vi "Program.vi"() -> ()   [LabVIEW 2014]
panel:
  in  "stop":bool
  out "error out":errorcluster
  in  "error in (no error)":errorcluster
  in  "设置":bool
  out "转速方向":bool
  out "转矩方向":bool
  in  "停机":bool
  out "欠压":bool
  out "过压":bool
  out "过流":bool
  out "过速":bool
  out "模块过温":bool
  out "电机过温":bool
  out "开关错误":bool
  out "模块故障":bool
  out "String":string
  in  "参数3":dbl
  in  "参数2":dbl
  in  "参数1":dbl
  in  "指令名":dbl
  in  "发送":bool
  in  "录波?L":bool caption="录波"
  out "波形文件大小L":string
  out "已录波L":string
  out "录波开始时间L":string
  in  "模式选择L":u16(ring) items=["示波模式", "录波模式", "XY图模式"]
  out "XY Graph L":cluster{"Y":dbl[], "Y":dbl[]}[](graph)
  in  "Choose 2":u16(ring) items=["Estlalpha", "AlphaErr", "speed", "iq", "id"]
  in  "Choose 1":u16(ring) items=["Estlalpha", "AlphaErr", "speed", "iq", "id"]
  in  "时频域转换 2":bool
  out "Graph 2":dbl[](graph)
  in  "时频域转换 1":bool
  out "Graph 1":dbl[](graph)
  in  "录波?R":bool caption="录波"
  out "波形文件大小R":string
  out "已录波R":string
  out "录波开始时间R":string
  in  "模式选择R":u16(ring) items=["示波模式", "录波模式", "XY图模式"]
  out "XY Graph R":cluster{"Y":dbl[], "Y":dbl[]}[](graph)
  in  "Choose 4":u16(ring) items=["Estlalpha", "AlphaErr", "speed", "iq", "id"]
  in  "Choose 3":u16(ring) items=["Estlalpha", "AlphaErr", "speed", "iq", "id"]
  in  "时频域转换 4":bool
  out "Graph 4":dbl[](graph)
  in  "时频域转换 3":bool
  out "Graph 3":dbl[](graph)
  # "电机工作状态"
  # "电机故障状态"
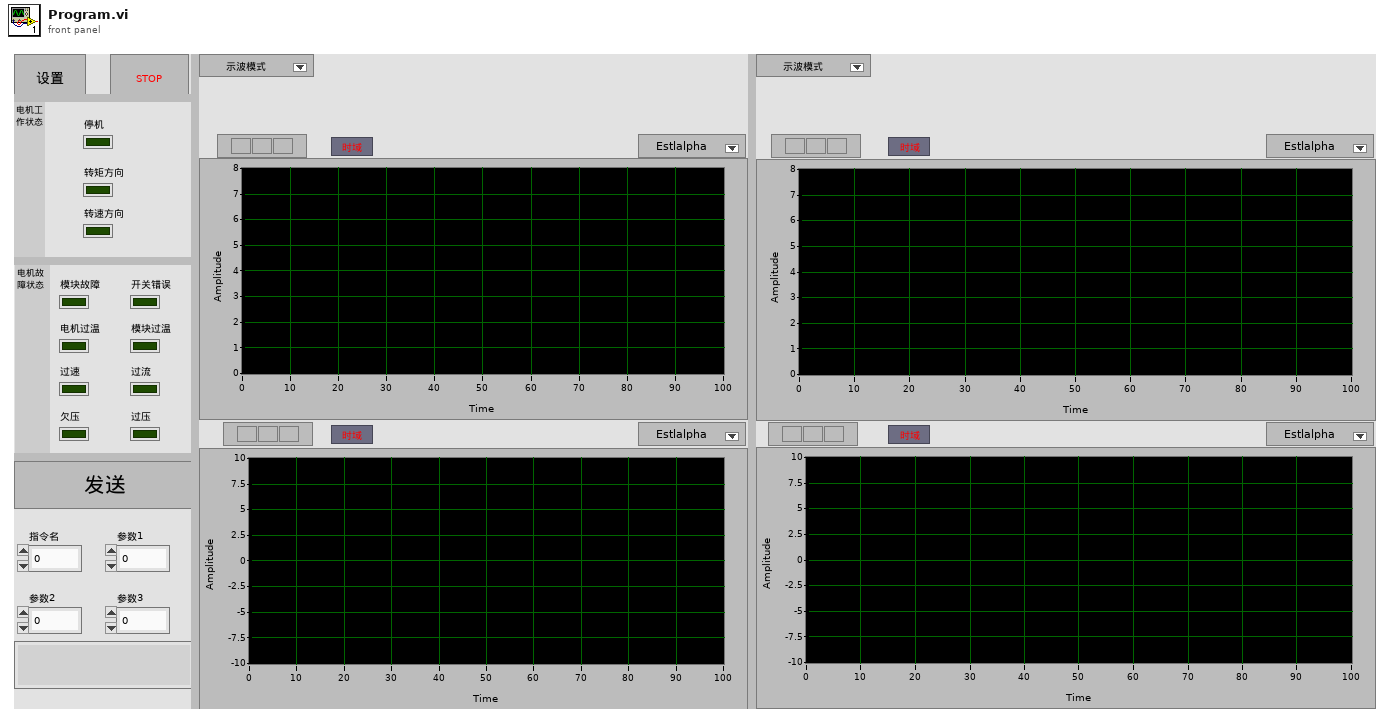
[diagram p1: front panel]
types:
  T1 = cluster{"ID":u32, "TimeStamp":u32, "TimeFlag":u8, "SendType":u8, "RemoteFlag":u8, "ExternFlag":u8, "DataLen":u8, "Data 0":u8, "Data 1":u8, "Data 2":u8, "Data 3":u8, "Data 4":u8, "Data 5":u8, "Data 6":u8, "Data 7":u8, "Reserved 0":u8, "Reserved 1":u8, "Reserved 2":u8}
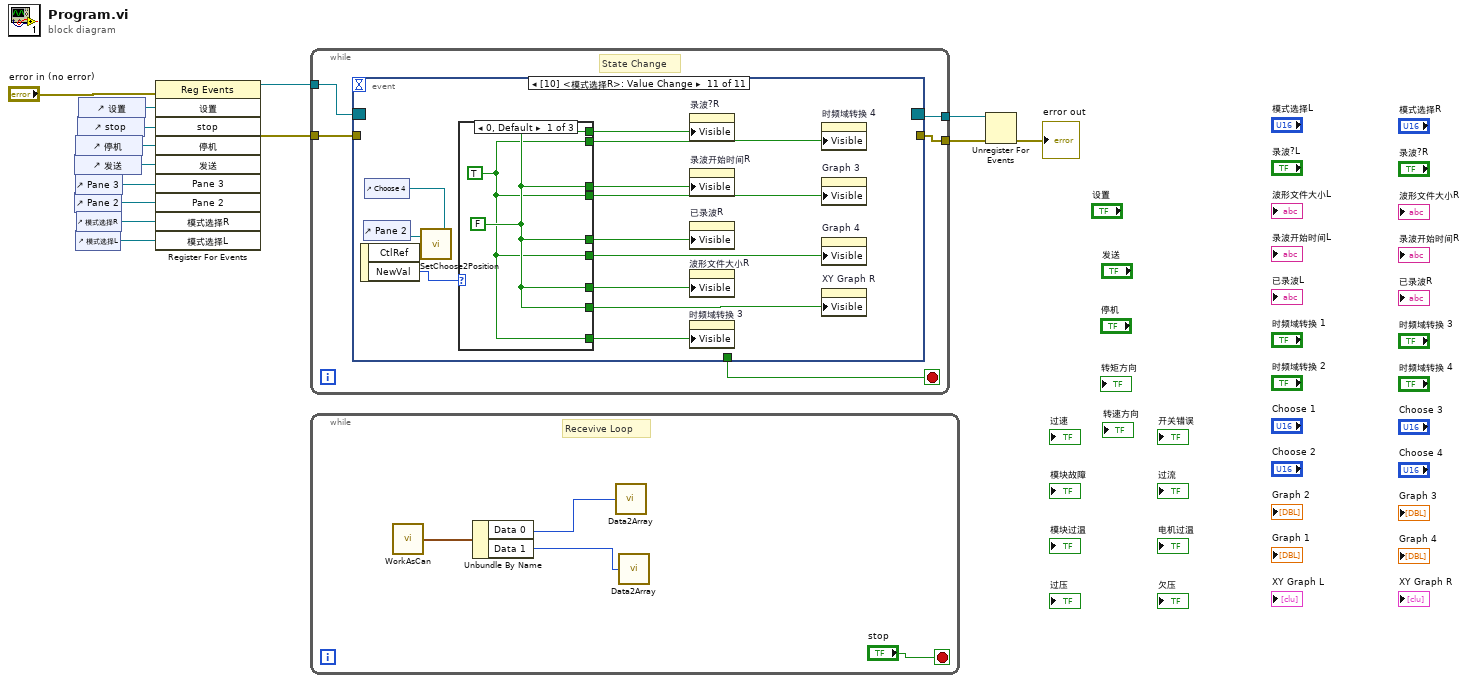
[diagram p0: block diagram]
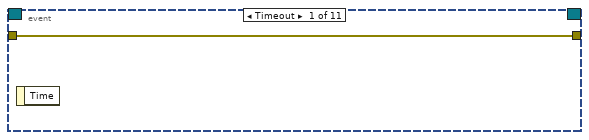
[diagram p2: hidden frame]
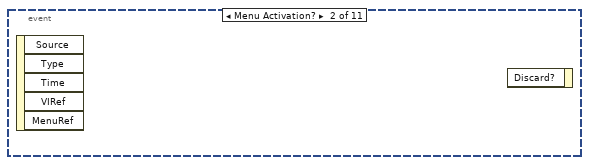
[diagram p3: hidden frame]
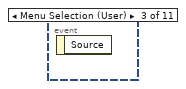
[diagram p4: hidden frame]
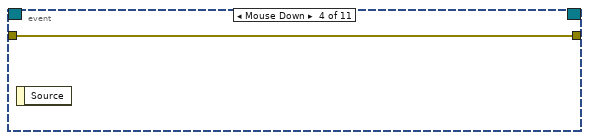
[diagram p5: hidden frame]
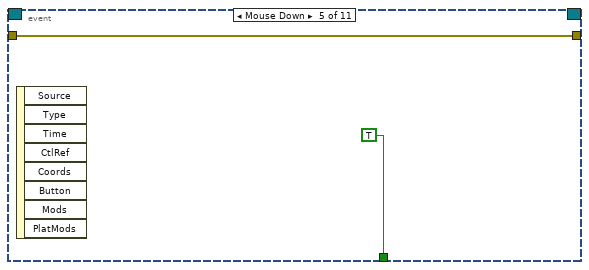
[diagram p6: hidden frame]
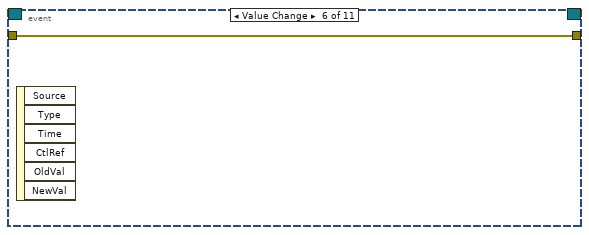
[diagram p7: hidden frame]
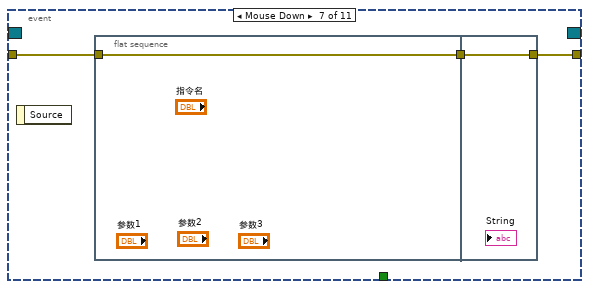
[diagram p8: hidden frame]
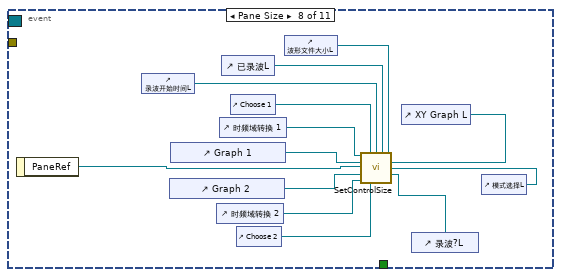
[diagram p9: hidden frame]
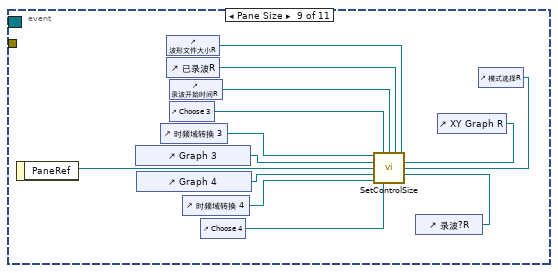
[diagram p10: hidden frame]
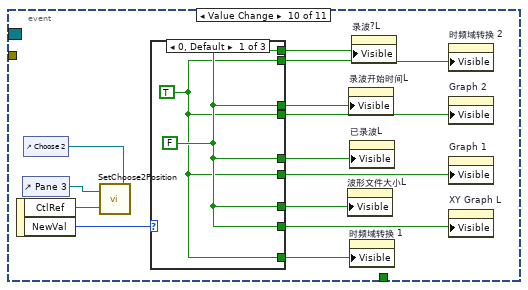
[diagram p11: hidden frame]
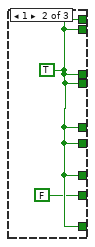
[diagram p12: hidden frame]
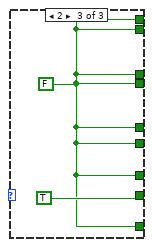
[diagram p13: hidden frame]
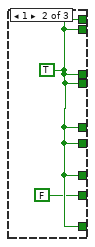
[diagram p14: hidden frame]
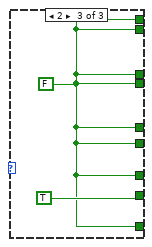
[diagram p15: hidden frame]
diagram:
  n1 = control-ref of="发送"() -> (w10:refnum<vi>)
  n2 = control-ref of="Pane 2"() -> (w3:refnum<vi>)
  n3 = control-ref of="停机"() -> (w11:refnum<vi>)
  n4 = control-ref of="Pane 3"() -> (w4:refnum<vi>)
  n5 = control-ref of="模式选择L"() -> (w1:refnum<vi>)
  n6 = control-ref of="模式选择R"() -> (w2:refnum<vi>)
  n7 = control-ref of="stop"() -> (w5:refnum<vi>)
  n8 = control-ref of="设置"() -> (w14:refnum<vi>)
  n9 = register-events(error in="error in (no error)", w14, w5, w11, w10, w4, w3, w2, w1) -> (reference out=w13:refnum<event-registration>, error out=w8:errorcluster)  [unwired: 1 in]
  n10 = while {
    tunnel: w13 -> [w19]
    tunnel: [w18] -> w12
    tunnel: w8 -> [w16]
    tunnel: [w15] -> w7
    stop <- w17 stop-if-true
    # "State Change"
    n11 = event shown="[10] <模式选择R>: Value Change" {
      selector: w19 -> [_ _ _ _ _ _ _ _ _ _ _]
      dyn-events: [_ _ _ _ _ _ _ _ _ _ _] -> w18
      timeout: _ -> [_ _ _ _ _ _ _ _ _ _ _]
      tunnel: [_ _ _ _ TRUE _ _ _ _ _ _] -> w17
      tunnel: w16 -> [w20 _ _ w21 w22 w24 w27 _ _ _ _]
      tunnel: [w20 _ _ w21 w22 w24 w25 _ _ _ _] -> w15
      event Timeout {
        n12 = event-data() -> ()  [unwired: 1 in, 1 out]
      }
      event Menu Activation? {
        n13 = event-data() -> ()  [unwired: 1 in, 5 out]
        n14 = event-data() -> ()  [unwired: 2 in, 1 out]
      }
      event Menu Selection (User) {
        n15 = event-data() -> ()  [unwired: 1 in, 1 out]
      }
      event Mouse Down {
        n16 = event-data() -> ()  [unwired: 1 in, 1 out]
      }
      event Mouse Down {
        n17 = event-data() -> ()  [unwired: 1 in, 8 out]
      }
      event Value Change {
        n18 = event-data() -> ()  [unwired: 1 in, 6 out]
      }
      event Mouse Down {
        n19 = event-data() -> ()  [unwired: 1 in, 1 out]
        n20 = flat-sequence {
          tunnel: w27 -> [w28]
          tunnel: [w28] -> w26
          tunnel: w26 -> [w29]
          tunnel: [w29] -> w25
          frame #0 {
          }
          frame #1 {
          }
        }
      }
      event Pane Size {
        n21 = event-data() -> ("PaneRef"=w31:refnum<vi>)  [unwired: 1 in]
        n22 = control-ref of="录波开始时间L"() -> (w36:refnum<vi>)
        n23 = control-ref of="Graph 2"() -> (w41:refnum<vi>)
        n24 = control-ref of="Graph 1"() -> (w42:refnum<vi>)
        n25 = control-ref of="时频域转换 2"() -> (w40:refnum<vi>)
        n26 = control-ref of="时频域转换 1"() -> (w39:refnum<vi>)
        n27 = control-ref of="已录波L"() -> (w35:refnum<vi>)
        n28 = control-ref of="Choose 1"() -> (w37:refnum<vi>)
        n29 = control-ref of="Choose 2"() -> (w38:refnum<vi>)
        n30 = control-ref of="波形文件大小L"() -> (w34:refnum<vi>)
        n31 = control-ref of="XY Graph L"() -> (w32:refnum<vi>)
        n32 = control-ref of="录波?L"() -> (w33:refnum<vi>)
        n33 = control-ref of="模式选择L"() -> (w30:refnum<vi>)
        n34 = call "SetControlSize.vi"("时频域1"=w39, "Choose1"=w37, "录波开始时间"=w36, "已录波"=w35, "录波文件大小"=w34, "Graph1"=w42, "XYGraph"=w32, "Pane Refnum"=w31, "Mode"=w30, "Graph2"=w41, "录波？"=w33, "时频域2"=w40, "Choose2"=w38) -> ()  [unwired: 3 in]
      }
      event Pane Size {
        n35 = event-data() -> ("PaneRef"=w55:refnum<vi>)  [unwired: 1 in]
        n36 = control-ref of="Graph 3"() -> (w54:refnum<vi>)
        n37 = control-ref of="Graph 4"() -> (w53:refnum<vi>)
        n38 = control-ref of="时频域转换 3"() -> (w51:refnum<vi>)
        n39 = control-ref of="波形文件大小R"() -> (w46:refnum<vi>)
        n40 = control-ref of="已录波R"() -> (w47:refnum<vi>)
        n41 = control-ref of="录波开始时间R"() -> (w48:refnum<vi>)
        n42 = control-ref of="Choose 3"() -> (w49:refnum<vi>)
        n43 = control-ref of="时频域转换 4"() -> (w52:refnum<vi>)
        n44 = control-ref of="Choose 4"() -> (w50:refnum<vi>)
        n45 = control-ref of="录波?R"() -> (w45:refnum<vi>)
        n46 = control-ref of="XY Graph R"() -> (w43:refnum<vi>)
        n47 = control-ref of="模式选择R"() -> (w44:refnum<vi>)
        n48 = call "SetControlSize.vi"("时频域1"=w51, "Choose1"=w49, "录波开始时间"=w48, "已录波"=w47, "录波文件大小"=w46, "Graph1"=w54, "XYGraph"=w43, "Pane Refnum"=w55, "Mode"=w44, "Graph2"=w53, "录波？"=w45, "时频域2"=w52, "Choose2"=w50) -> ()  [unwired: 3 in]
      }
      event Value Change {
        n49 = event-data() -> ("CtlRef"=w67:refnum<vi>, "NewVal"=w65:u16)  [unwired: 1 in]
        n50 = control-ref of="Pane 3"() -> (w68:refnum<vi>)
        n51 = control-ref of="Choose 2"() -> (w66:refnum<vi>)
        n52 = call "SetChoose2Position.vi"("Choose2"=w66, "Mode"=w67, "Pane Refnum"=w68) -> ()
        n53 = case shown="0, Default" w65 {
          tunnel: [w70 w72 w73] -> w64
          tunnel: [w69 w72 w73] -> w63
          tunnel: [w70 w72 w73] -> w62
          tunnel: [w69 w72 w73] -> w61
          tunnel: [w70 w72 w73] -> w60
          tunnel: [w69 w72 w73] -> w59
          tunnel: [w70 w72 w73] -> w58
          tunnel: [w70 FALSE TRUE] -> w57
          tunnel: [w69 w72 w73] -> w56
          frame 0, Default {
            w70 = FALSE
            w69 = TRUE
          }
          frame 1 {
            w72 = TRUE
          }
          frame 2 {
            w73 = FALSE
          }
        }
        n54 = property on="波形文件大小L" class="Str"("Visible"=w58) -> ()  [unwired: 2 in, 2 out]
        n55 = property on="录波开始时间L" class="Str"("Visible"=w62) -> ()  [unwired: 2 in, 2 out]
        n56 = property on="已录波L" class="Str"("Visible"=w60) -> ()  [unwired: 2 in, 2 out]
        n57 = property on="时频域转换 1" class="Bool (strict)"("Visible"=w56) -> ()  [unwired: 2 in, 2 out]
        n58 = property on="录波?L" class="Bool (strict)"("Visible"=w64) -> ()  [unwired: 2 in, 2 out]
        n59 = property on="时频域转换 2" class="Bool (strict)"("Visible"=w63) -> ()  [unwired: 2 in, 2 out]
        n60 = property on="Graph 2" class="WFGraph (strict)"("Visible"=w61) -> ()  [unwired: 2 in, 2 out]
        n61 = property on="Graph 1" class="WFGraph (strict)"("Visible"=w59) -> ()  [unwired: 2 in, 2 out]
        n62 = property on="XY Graph L" class="XYGraph (strict)"("Visible"=w57) -> ()  [unwired: 2 in, 2 out]
      }
      event Value Change {
        n63 = event-data() -> ("CtlRef"=w86:refnum<vi>, "NewVal"=w84:u16)  [unwired: 1 in]
        n64 = control-ref of="Pane 2"() -> (w87:refnum<vi>)
        n65 = control-ref of="Choose 4"() -> (w85:refnum<vi>)
        n66 = call "SetChoose2Position.vi"("Choose2"=w85, "Mode"=w86, "Pane Refnum"=w87) -> ()
        n67 = case shown="0, Default" w84 {
          tunnel: [w89 w91 w92] -> w83
          tunnel: [w88 w91 w92] -> w82
          tunnel: [w89 w91 w92] -> w81
          tunnel: [w88 w91 w92] -> w80
          tunnel: [w89 w91 w92] -> w79
          tunnel: [w88 w91 w92] -> w78
          tunnel: [w89 w91 w92] -> w77
          tunnel: [w89 FALSE TRUE] -> w76
          tunnel: [w88 w91 w92] -> w75
          frame 0, Default {
            w89 = FALSE
            w88 = TRUE
          }
          frame 1 {
            w91 = TRUE
          }
          frame 2 {
            w92 = FALSE
          }
        }
        n68 = property on="录波?R" class="Bool (strict)"("Visible"=w83) -> ()  [unwired: 2 in, 2 out]
        n69 = property on="录波开始时间R" class="Str"("Visible"=w81) -> ()  [unwired: 2 in, 2 out]
        n70 = property on="已录波R" class="Str"("Visible"=w79) -> ()  [unwired: 2 in, 2 out]
        n71 = property on="波形文件大小R" class="Str"("Visible"=w77) -> ()  [unwired: 2 in, 2 out]
        n72 = property on="时频域转换 3" class="Bool (strict)"("Visible"=w75) -> ()  [unwired: 2 in, 2 out]
        n73 = property on="时频域转换 4" class="Bool (strict)"("Visible"=w82) -> ()  [unwired: 2 in, 2 out]
        n74 = property on="Graph 3" class="WFGraph (strict)"("Visible"=w80) -> ()  [unwired: 2 in, 2 out]
        n75 = property on="Graph 4" class="WFGraph (strict)"("Visible"=w78) -> ()  [unwired: 2 in, 2 out]
        n76 = property on="XY Graph R" class="XYGraph (strict)"("Visible"=w76) -> ()  [unwired: 2 in, 2 out]
      }
    }
  }
  n77 = while {
    stop <- "stop" stop-if-true
    # "Recevive Loop"
    n78 = call "WorkAsCan.vi"() -> ("VCI_CAN_OBJ 2"=w96:T1)  [unwired: 2 in]
    n79 = Unbundle By Name(w96) -> ("Data 0"=w95:u8, "Data 1"=w94:u8)
    n80 = call "Data2Array.vi"("date"=w95) -> ()  [unwired: 4 in, 1 out]
    n81 = call "Data2Array.vi"("date"=w94) -> ()  [unwired: 4 in, 1 out]
  }
  n82 = Unregister For Events(event registration refnum=w12, error in=w7) -> (error out=→"error out":errorcluster)
